vi "Cast Data to Log.vi"(4 "Data in":T1={"Closed Loop Enabled"=FALSE, "Proportional valve 1"=0.0, "Proportional valve 2"=0.0, "Controller"={"Control Algorithm"=enum."LQG-LTR", "K"={"A"=[[1.62451, -0.722865, 0.589162, 0.0258055, -0.291247, -0.19871], [0.616764, 0.243215, 0.627021, 0.310989, -0.690401, -0.192347], [-1.01378, 1.19782, 0.595116, 0.307107, -0.873915, -0.221858], [0.460934, 0.301624, 0.892121, 0.145562, -1.07734, -0.276248], [-0.148448, 0.409634, 0.289356, 0.289437, -0.348463, -0.146062], [-0.46568, 0.0291416, 0.0291565, 0.00664228, 0.274253, 0.0367555]], "B"=[[-0.400941, 1.75732], [-0.839249, -0.493575], [-1.18504, -0.379909], [-0.825179, 0.0646258], [0.655259, -0.107787], [0.351957, -0.140832]], "C"=[[0.185781, 0.5585, 1.12711, -0.0910001, -2.59125, -0.578566], [-1.86119, 1.94847, -1.12933, 0.309409, -0.22228, -0.226668]], "D"=[[4.45609, -0.0220273], [-0.0283496, 4.51922]]}, "PI/W1"={"A"=[[-4.94989, 0.0218181, -352.966, 23.8192, -3.10685, -0.000952287], [-0.0218181, -4.904857, 23.4819, -343.472, 0.000977323, -3.58066], [0.0389045, 0.0, -31.6573, 0.0287797, 0.0245405, 0.0], [0.0, 0.0381972, 0.0287797, -31.6573, 0.0, 0.0280468], [0.0, 0.0325383, 0.0240248, -0.0293675, -0.0245405, 0.0], [0.031831, 0.0, -0.0282058, 0.0, 0.0, 0.0]], "B"=[[28.0692, -23.9099], [-23.3912, 28.5852], [31.6468, -0.0287797], [-0.0287797, 31.6468], [-0.0282058, -0.0293675], [0.0282058, -0.0240214]], "C"=[[4.94989, 0.0218181, 314.896, 0.0907351, 3.10685, 0.000952287], [10.0218181, 4.90457, -0.0906726, 314.884, -0.000977323, 3.58066]], "D"=[[0.0, 0.0], [0.0, 0.0]]}, "W2"={"A"=[[-4.94989, 0.0218181, -352.966, 23.8192, -3.10685, -0.000952287], [-0.0218181, -4.904857, 23.4819, -343.472, 0.000977323, -3.58066], [0.0389045, 0.0, -31.6573, 0.0287797, 0.0245405, 0.0], [0.0, 0.0381972, 0.0287797, -31.6573, 0.0, 0.0280468], [0.0, 0.0325383, 0.0240248, -0.0293675, -0.0245405, 0.0], [0.031831, 0.0, -0.0282058, 0.0, 0.0, 0.0]], "B"=[[28.0692, -23.9099], [-23.3912, 28.5852], [31.6468, -0.0287797], [-0.0287797, 31.6468], [-0.0282058, -0.0293675], [0.0282058, -0.0240214]], "C"=[[4.94989, 0.0218181, 314.896, 0.0907351, 3.10685, 0.000952287], [10.0218181, 4.90457, -0.0906726, 314.884, -0.000977323, 3.58066]], "D"=[[0.0, 0.0], [0.0, 0.0]]}}, "Setpoint"={"Setpoints"={"Setpoint Tank 1"=0.0, "Setpoint Tank 2"=0.0, "Sin on-off"=enum."On", "Amplitude Tank 1"=0.0, "Amplitude Tank 2"=0.0, "Frequency Tank 1"=0.0, "Frequency Tank 2"=0.0, "Phase Tank 1"=0.0, "Phase Tank 2"=0.0}, "Disturbance"={"Distubance pump 1"=FALSE, "Amplitude Pump 1"=0.0, "Distubance pump 2"=FALSE, "Amplitude Pump 2"=0.0}}, "Plant Control Variables"={"Tank 1 Level"=0.0, "Tank 2 Level"=0.0, "Tank 3 Level"=0.0, "Tank 4 Level"=0.0, "Pump 1"=0.0, "Pump 2"=0.0, "Setpoint 1 signal"=0.0, "Setpoint 2 signal"=0.0}}) -> (1 "Data out":dbl[](array[numeric]))   [LabVIEW 2020]
uses:
  Real-Time/controls/Controller Data.ctl
  Real-Time/Control Algorithm/Control Algorithm Data.ctl
  Real-Time/Control Algorithm/Control Algorithm Selection.ctl
  controls/Setpoints.ctl
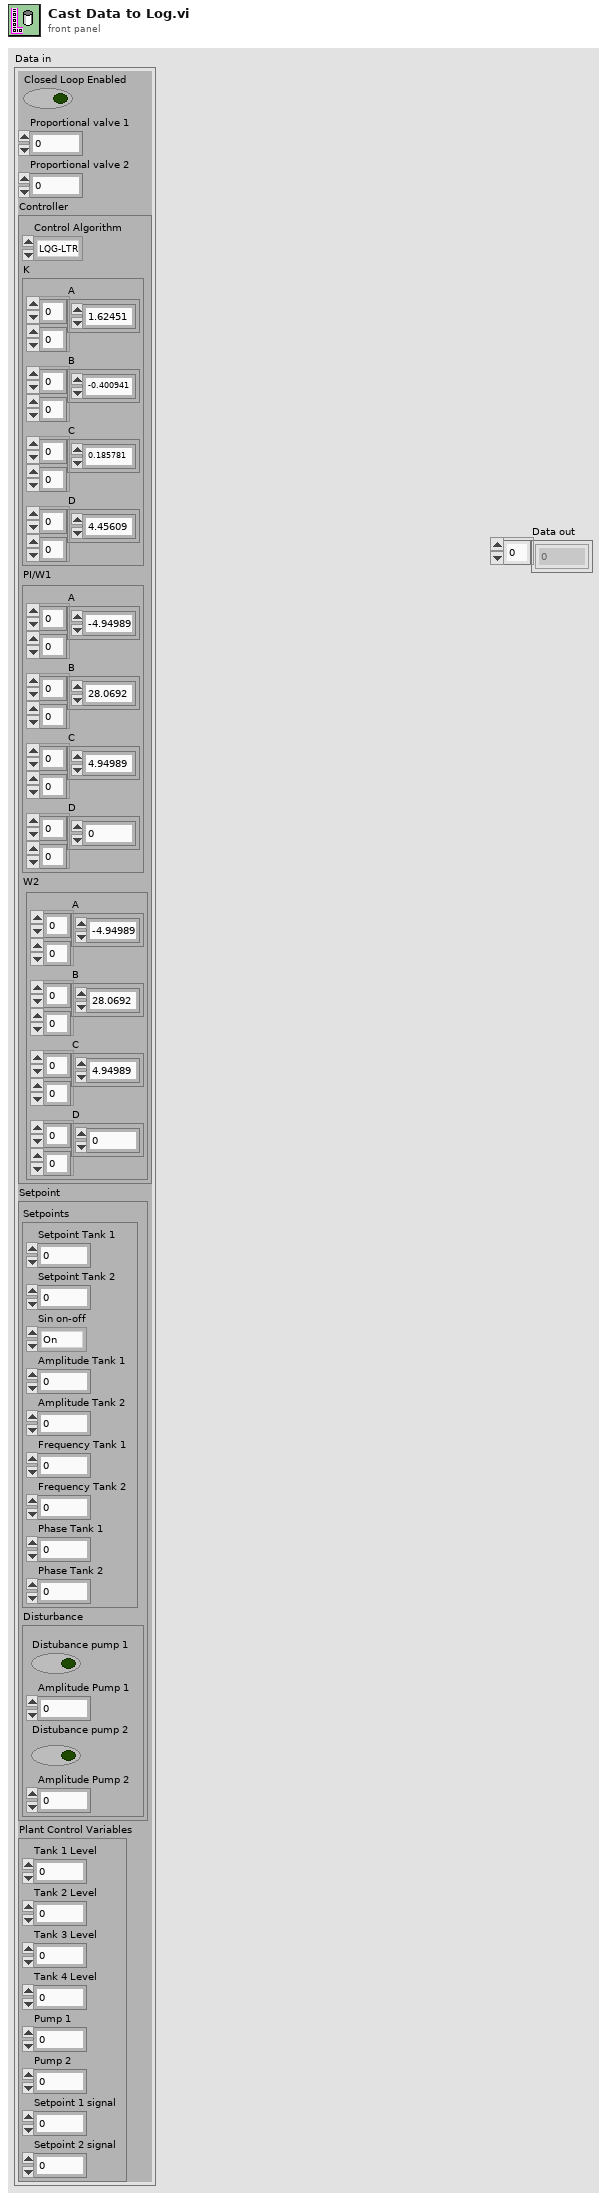
[diagram p1: front panel]
types:
  T1 = typedef "Controller Data.ctl" = cluster{"Closed Loop Enabled":bool, "Proportional valve 1":dbl, "Proportional valve 2":dbl, "Controller":T2, "Setpoint":T4, "Plant Control Variables":cluster{"Tank 1 Level":dbl, "Tank 2 Level":dbl, "Tank 3 Level":dbl, "Tank 4 Level":dbl, "Pump 1":dbl, "Pump 2":dbl, "Setpoint 1 signal":dbl, "Setpoint 2 signal":dbl}}
  T2 = typedef "Control Algorithm Data.ctl" = cluster{"Control Algorithm":T3, "K":cluster{"A":dbl[][], "B":dbl[][], "C":dbl[][], "D":dbl[][]}, "PI/W1":cluster{"A":dbl[][], "B":dbl[][], "C":dbl[][], "D":dbl[][]}, "W2":cluster{"A":dbl[][], "B":dbl[][], "C":dbl[][], "D":dbl[][]}}
  T3 = typedef "Control Algorithm Selection.ctl" = enum16{"LQG-LTR", "Hinf", "New Controller"}
  T4 = typedef "Setpoints.ctl" = cluster{"Setpoints":cluster{"Setpoint Tank 1":dbl, "Setpoint Tank 2":dbl, "Sin on-off":enum32{"On", "Off"}, "Amplitude Tank 1":dbl, "Amplitude Tank 2":dbl, "Frequency Tank 1":dbl, "Frequency Tank 2":dbl, "Phase Tank 1":dbl, "Phase Tank 2":dbl}, "Disturbance":cluster{"Distubance pump 1":bool, "Amplitude Pump 1":dbl, "Distubance pump 2":bool, "Amplitude Pump 2":dbl}}
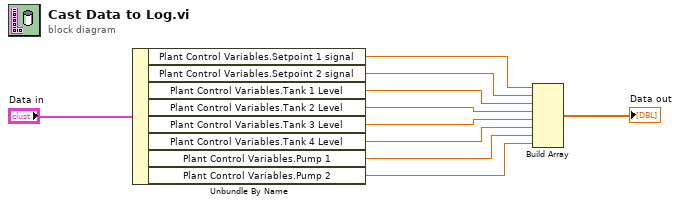
[diagram p0: block diagram]
diagram:
  n1 = Unbundle By Name("Data in") -> ("Plant Control Variables.Setpoint 1 signal"=w3:dbl, "Plant Control Variables.Setpoint 2 signal"=w2:dbl, "Plant Control Variables.Tank 1 Level"=w10:dbl, "Plant Control Variables.Tank 2 Level"=w9:dbl, "Plant Control Variables.Tank 3 Level"=w8:dbl, "Plant Control Variables.Tank 4 Level"=w7:dbl, "Plant Control Variables.Pump 1"=w6:dbl, "Plant Control Variables.Pump 2"=w5:dbl)
  n2 = Build Array(w3, w2, w10, w9, w8, w7, w6, w5) -> (→"Data out":dbl[])
